vi "event_interface_load_subpanel.vi"(6 "event_interface":refnum<user-event>, 8 "error in (no error)":errorcluster, 11 "interface":T1) -> (0 "error out":errorcluster)   [LabVIEW 2015, in "lv-interface-dom-nre.lvlib"]
uses:
  lv-interface-dom-nre.lvlib
  _controls/event_interface.ctl
  _controls/event_interface_command.ctl
  lv-interface-sub-common/_controls/interface_selection.ctl
  lv-interface-sub-common/lv-interface-sub-common.lvlib
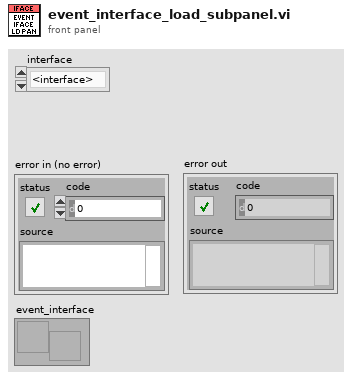
[diagram p1: front panel]
types:
  T1 = typedef "lv-interface-sub-common.lvlib/interface_selection.ctl" = enum16{"<interface>", "sub_interface_1", "sub_interface_2", "<null>"}
  T2 = typedef "lv-interface-dom-nre.lvlib/event_interface_command.ctl" = enum16{"<event_interface_cmd>", "defer_panel_updates", "undefer_panel_updates", "load_interface", "<null>"}
  T3 = typedef "lv-interface-dom-nre.lvlib/event_interface.ctl" = cluster{"command":T2, "data":variant}
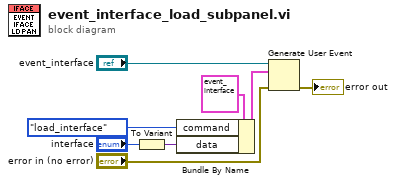
[diagram p0: block diagram]
diagram:
  n1 = To Variant(anything="interface") -> (Variant=w1:variant)
  n2 = Bundle By Name(cluster=T3 {"command"=enum."<event_interface_cmd>", "data"=variant} ("event data"), "command"=event_interface_command."load_interface", "data"=w1) -> (w6:T3)
  n3 = Generate User Event(user event="event_interface", event data cluster=w6, error in="error in (no error)") -> (error out=→"error out":errorcluster)  [unwired: 1 in, 1 out]
